vi "Actor Core.vi"(8 "error in":errorcluster, 11 "Nested in":refnum<class "Calling Actor.lvclass">) -> (0 "error out":errorcluster, 3 "Actor out":refnum<class "Actor.lvclass">)   [LabVIEW 2020, in "Calling Actor.lvlib" / "Calling Actor.lvclass"]
doc: "(<B>Filename</B>: Actor Framework.lvlib:Actor.lvclass:Actor Core.vi)\n\nReceives messages to the actor, reacts to them, and initiates any error handling that may shut the actor down.\n\nDescendant classes may override this VI to append parallel tasks for the actor to complete while it handles messages. Overrides use the Call Parent Method node."
uses:
  Calling Actor.lvclass
  C:/Program Files (x86)/National Instruments/LabVIEW 2020/vi.lib/ActorFramework/Actor/Actor.lvclass
  <vilib>/ActorFramework/Actor/Actor.lvclass
  Nested Actor/Nested Actor.lvclass
  Nested Actor/Actor Type.ctl
  Calling Actor Messages/Perform Slow Buffer Task Msg/Perform Slow Buffer Task Msg.lvclass
  C:/Users/Thomas.McQuillan/Desktop/deleteme/Buffer Question/Nested Actor Messages/Abstract Message Msg/Abstract Message Msg.lvclass
  Calling Actor Messages/Perform Fast Buffer Task Msg/Perform Fast Buffer Task Msg.lvclass
  Nested Actor/Nested Actor.lvclass/Nested Actor.ctl
  <vilib>/ActorFramework/Actor/Actor.lvclass/Actor.ctl
  <vilib>/ActorFramework/Message Enqueuer/Message Enqueuer.lvclass/Message Enqueuer.ctl
  Calling Actor.lvclass/Calling Actor.ctl
  <vilib>/ActorFramework/Message Enqueuer/Init from Existing Queue.vi
  <vilib>/ActorFramework/Message Enqueuer/Enqueue.vi
  <vilib>/ActorFramework/Stop Msg/Stop Msg.lvclass
  C:/Program Files (x86)/National Instruments/LabVIEW 2020/vi.lib/ActorFramework/Message/Message.lvclass
  <vilib>/ActorFramework/Message Priority Queue/Priority Enqueue.vi
  <vilib>/ActorFramework/Message Enqueuer/Message Enqueuer.lvclass
types:
  T1 = typedef "Nested Actor.lvlib/Nested Actor.lvclass/Actor Type.ctl" = enum16{"Slow Buffer", "Fast Buffer"}
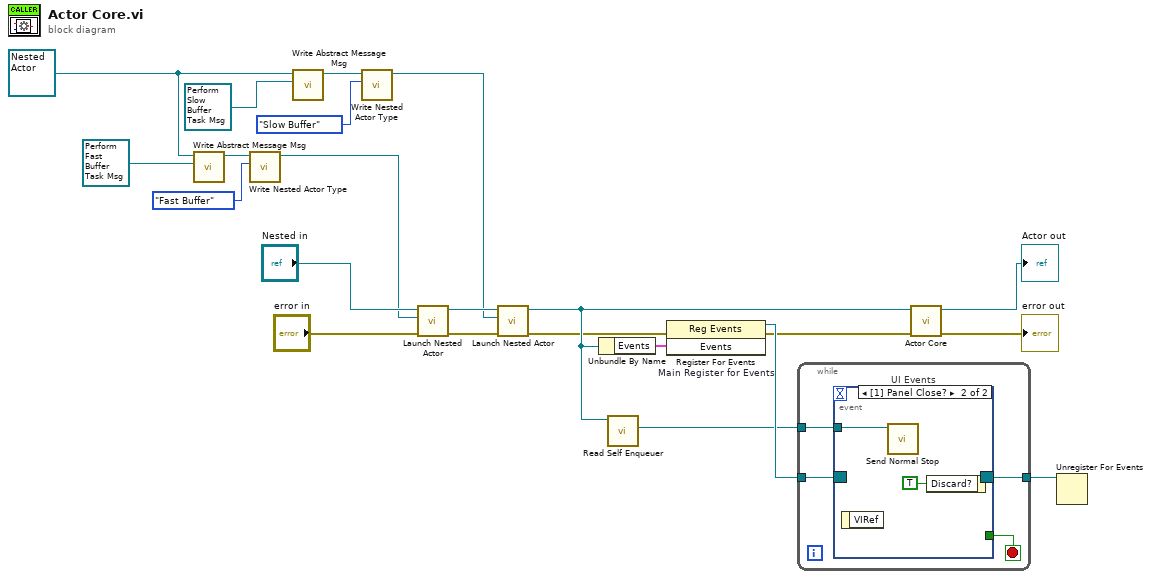
[diagram p0: block diagram]
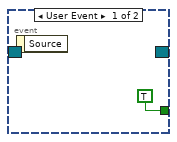
[diagram p2: hidden frame]
diagram:
  w3 = refnum<class "Nested Actor.lvclass"> refnum ("Nested Actor.lvlib:Nested Actor.lvclass")
  n1 = call "Write Abstract Message Msg.vi"("Nested Actor.lvlib:Abstract Message Msg.lvclass"=refnum<class "Perform Fast Buffer Task Msg.lvclass"> refnum ("Calling Actor.lvlib:Perform Fast Buffer Task Msg.lvclass"), "Nested Actor in"=w3) -> ("Nested Actor out"=w2:refnum<class "Nested Actor.lvclass">)  [unwired: 9 in]
  n2 = call "Write Nested Actor Type.vi"("Nested Actor Type"=Actor_Type."Fast Buffer", "Nested Actor in"=w2) -> ("Nested Actor out"=w9:refnum<class "Nested Actor.lvclass">)  [unwired: 9 in]
  n3 = call "Write Abstract Message Msg.vi"("Nested Actor.lvlib:Abstract Message Msg.lvclass"=refnum<class "Perform Slow Buffer Task Msg.lvclass"> refnum ("Calling Actor.lvlib:Perform Slow Buffer Task Msg.lvclass"), "Nested Actor in"=w3) -> ("Nested Actor out"=w5:refnum<class "Nested Actor.lvclass">)  [unwired: 9 in]
  n4 = call "Write Nested Actor Type.vi"("Nested Actor Type"=Actor_Type."Slow Buffer", "Nested Actor in"=w5) -> ("Nested Actor out"=w8:refnum<class "Nested Actor.lvclass">)  [unwired: 9 in]
  n5 = call <vilib>:"Launch Nested Actor.vi"("error in (no error)"="error in", "Nested Actor"=w9, "Caller Actor in"="Nested in") -> ("error out"=w13:errorcluster, "Caller Actor out"=w14:refnum<class "Calling Actor.lvclass">)  [unwired: 6 in, 1 out]
  n6 = call <vilib>:"Launch Nested Actor.vi"("error in (no error)"=w13, "Nested Actor"=w8, "Caller Actor in"=w14) -> ("error out"=w10:errorcluster, "Caller Actor out"=w11:refnum<class "Calling Actor.lvclass">)  [unwired: 6 in, 1 out]
  n7 = Unbundle By Name(w11) -> ("Events"=w19:cluster{"Stop":refnum<user-event>})
  n8 = call <vilib>:"Read Self Enqueuer.vi"("Actor"=w11) -> ("Self Enqueuer"=w17:refnum<class "Message Enqueuer.lvclass">)  [unwired: 10 in]
  n9 = register-events "Main Register for Events"(error in=w10, w19) -> (reference out=w20:refnum<event-registration>, error out=w16:errorcluster)  [unwired: 1 in]
  n10 = while {
    tunnel: w20 -> [w26]
    tunnel: [w24] -> w18
    tunnel: w17 -> [w23]
    stop <- w25 stop-if-true
    n11 = event "UI Events" shown="[1] Panel Close?" {
      selector: w26 -> [_ _]
      dyn-events: [_ _] -> w24
      timeout: _ -> [_ _]
      tunnel: [TRUE _] -> w25
      tunnel: w23 -> [_ w28]
      event User Event {
        n12 = event-data() -> ()  [unwired: 1 in, 1 out]
      }
      event Panel Close? {
        n13 = event-data() -> ()  [unwired: 1 in, 1 out]
        n14 = call <vilib>:"Send Normal Stop.vi"("Message Enqueuer"=w28) -> ()  [unwired: 10 in, 1 out]
        n15 = event-data("Discard?"=TRUE) -> ()  [unwired: 1 in, 1 out]
      }
    }
  }
  n16 = call-parent "Actor Core.vi"("error in"=w16, "Actor in"=w11) -> ("error out"=→"error out":errorcluster, "Actor out"=→"Actor out":refnum<class "Actor.lvclass">)  [unwired: 8 in]
  n17 = Unregister For Events(event registration refnum=w18) -> ()  [unwired: 1 in, 1 out]
